vi "Move X-Y to specific position.vi"(8 "error in (no error) 3":errorcluster, 10 "position 2":string, 11 "position 1":string) -> (0 "error out 3":errorcluster, 1 "cmd response 2":string, 2 "cmd response":string, 3 "Enable response":string, 4 "Finished moving":bool)   [LabVIEW 2016]
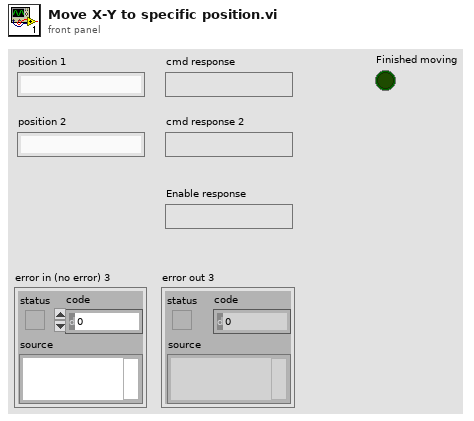
[diagram p1: front panel]
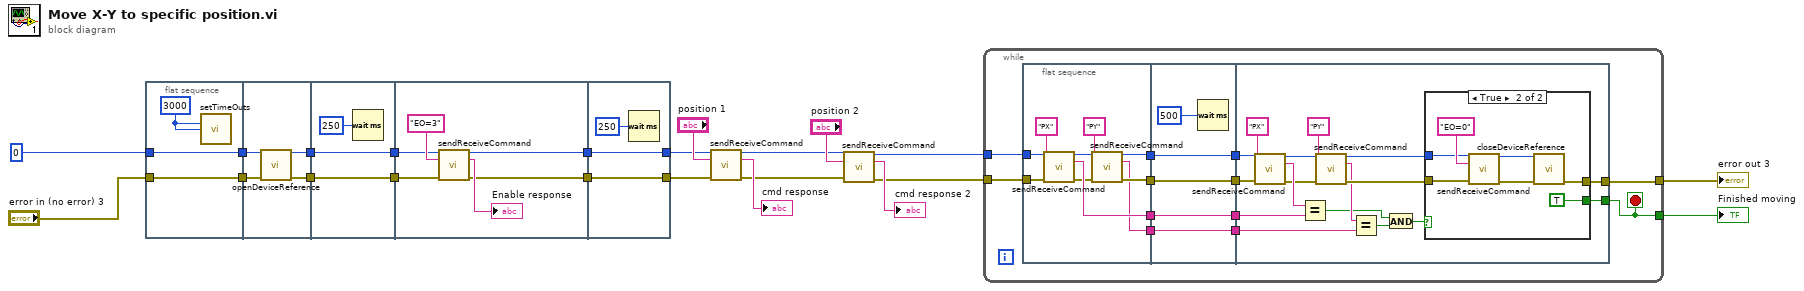
[diagram p0: block diagram]
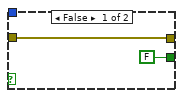
[diagram p2: hidden frame]
diagram:
  n1 = flat-sequence {
    tunnel: 0 -> [w24]
    tunnel: [w24] -> w18
    tunnel: "error in (no error) 3" -> [w23]
    tunnel: [w23] -> w17
    tunnel: w18 -> [w29]
    tunnel: w17 -> [w28]
    tunnel: [w27] -> w6
    tunnel: [w26] -> w5
    tunnel: w6 -> [w32]
    tunnel: w5 -> [w31]
    tunnel: [w32] -> w4
    tunnel: [w31] -> w3
    tunnel: w4 -> [w36]
    tunnel: w3 -> [w35]
    tunnel: [w34] -> w2
    tunnel: [w33] -> w1
    tunnel: [w40] -> w16
    tunnel: [w41] -> w20
    tunnel: w2 -> [w41]
    tunnel: w1 -> [w40]
    frame #0 {
      w25 = 3000 ("read_timeout")
      n2 = call "setTimeOuts.vi"("read_timeout (ms)"=w25, "write_timeout (ms)"=w25) -> ()  [unwired: 13 in, 1 out]
    }
    frame #1 {
      n3 = call "openDeviceReference.vi"("deviceIndex"=w29, "error in (no error)"=w28) -> ("reference"=w27:i32, "error out"=w26:errorcluster)  [unwired: 12 in]
    }
    frame #2 {
      n4 = Wait (ms)(milliseconds to wait=u32 250) -> ()  [unwired: 1 out]
    }
    frame #3 {
      n5 = call "sendReceiveCommand.vi"("reference (in)"=w36, "write_string"="EO=3" ("raw_cmd 2"), "error in (no error)"=w35) -> ("reference (out)"=w34:i32, "read_string"=→"Enable response":string, "error out"=w33:errorcluster)  [unwired: 10 in]
    }
    frame #4 {
      n6 = Wait (ms)(milliseconds to wait=u32 250) -> ()  [unwired: 1 out]
    }
  }
  n7 = call "sendReceiveCommand.vi"("reference (in)"=w20, "write_string"="position 1", "error in (no error)"=w16) -> ("reference (out)"=w13:i32, "read_string"=→"cmd response":string, "error out"=w12:errorcluster)  [unwired: 10 in]
  n8 = call "sendReceiveCommand.vi"("reference (in)"=w13, "write_string"="position 2", "error in (no error)"=w12) -> ("reference (out)"=w11:i32, "read_string"=→"cmd response 2":string, "error out"=w10:errorcluster)  [unwired: 10 in]
  n9 = while {
    tunnel: [w47] -> w8
    tunnel: w11 -> [w53]
    tunnel: w10 -> [w52]
    tunnel: [w42] -> w7
    stop <- w42 stop-if-true
    n10 = flat-sequence {
      tunnel: w53 -> [w62]
      tunnel: w52 -> [w61]
      tunnel: [w56] -> w51
      tunnel: [w55] -> w50
      tunnel: [w60] -> w45
      tunnel: [w54] -> w43
      tunnel: w51 -> [w68]
      tunnel: w50 -> [w67]
      tunnel: [w68] -> w49
      tunnel: [w67] -> w48
      tunnel: [w65] -> w46
      tunnel: w45 -> [w65]
      tunnel: [w64] -> w44
      tunnel: w43 -> [w64]
      tunnel: w49 -> [w84]
      tunnel: w48 -> [w83]
      tunnel: [w82] -> w47
      tunnel: [w81] -> w42
      tunnel: w46 -> [w79]
      tunnel: w44 -> [w71]
      frame #0 {
        n11 = call "sendReceiveCommand.vi"("reference (in)"=w62, "write_string"="PX" ("raw_cmd 2"), "error in (no error)"=w61) -> ("reference (out)"=w58:i32, "read_string"=w60:string, "error out"=w57:errorcluster)  [unwired: 10 in]
        n12 = call "sendReceiveCommand.vi"("reference (in)"=w58, "write_string"="PY" ("raw_cmd 2"), "error in (no error)"=w57) -> ("reference (out)"=w56:i32, "read_string"=w54:string, "error out"=w55:errorcluster)  [unwired: 10 in]
      }
      frame #1 {
        n13 = Wait (ms)(milliseconds to wait=500) -> ()  [unwired: 1 out]
      }
      frame #2 {
        n14 = call "sendReceiveCommand.vi"("reference (in)"=w84, "write_string"="PX" ("raw_cmd 2"), "error in (no error)"=w83) -> ("reference (out)"=w76:i32, "read_string"=w80:string, "error out"=w75:errorcluster)  [unwired: 10 in]
        n15 = Equal?(x=w80, y=w79) -> (x = y?=w69:bool)
        n16 = call "sendReceiveCommand.vi"("reference (in)"=w76, "write_string"="PY" ("raw_cmd 2"), "error in (no error)"=w75) -> ("reference (out)"=w74:i32, "read_string"=w70:string, "error out"=w73:errorcluster)  [unwired: 10 in]
        n17 = Equal?(x=w70, y=w71) -> (x = y?=w72:bool)
        n18 = And(x=w69, y=w72) -> (x .and. y?=w78:bool)
        n19 = case shown="True" w78 {
          tunnel: [w87 w94] -> w82
          tunnel: w73 -> [w87 w90]
          tunnel: w74 -> [_ w89]
          tunnel: [FALSE TRUE] -> w81
          frame False {
          }
          frame True {
            n20 = call "sendReceiveCommand.vi"("reference (in)"=w89, "write_string"="EO=0" ("raw_cmd 2"), "error in (no error)"=w90) -> ("reference (out)"=w92:i32, "error out"=w91:errorcluster)  [unwired: 10 in, 1 out]
            n21 = call "closeDeviceReference.vi"("reference"=w92, "error in (no error)"=w91) -> ("error out"=w94:errorcluster)  [unwired: 13 in]
          }
        }
      }
    }
  }
  "error out 3" <- w8
  "Finished moving" <- w7
